vi "雷达流速仪设置窗口.vi"() -> (3 "确定输出":bool)   [LabVIEW 2016, in "雷达流速仪.lvlib"]
panel:
  out "开关":bool
  in  "雷达流速仪类型":string(combo)
  in  "串口":refnum<visa-resource-name>="COM6"
  in  "雷达流速仪型号":string="LDH20-1QC"
  in  "确定":bool
  in  "取消":bool
  in  "串口开关":bool
  # "设置雷达流速仪参数"
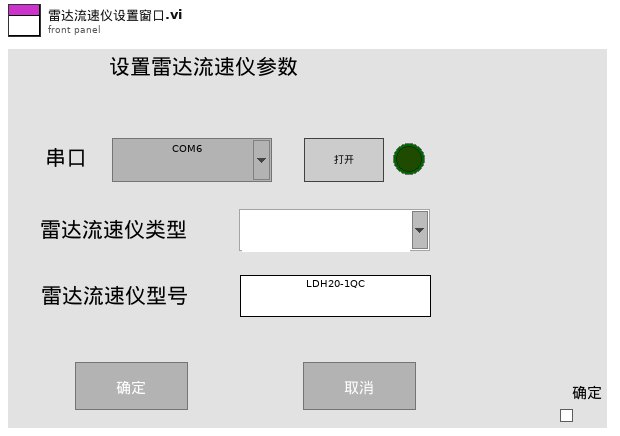
[diagram p1: front panel]
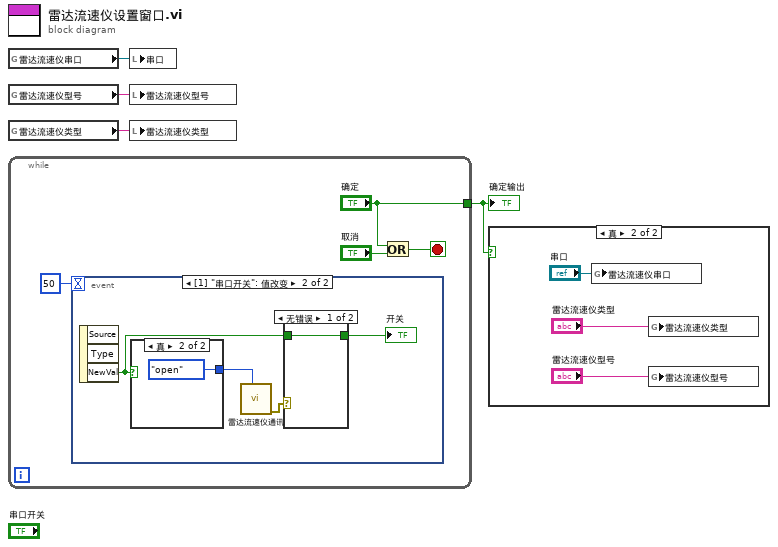
[diagram p0: block diagram]
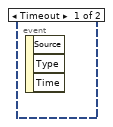
[diagram p3: hidden frame]
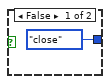
[diagram p5: hidden frame]
diagram:
  n1 = global read "雷达流速仪全局变量.vi" "雷达流速仪串口"() -> (w3:refnum<visa-resource-name>)
  n2 = global read "雷达流速仪全局变量.vi" "雷达流速仪型号"() -> (w2:string)
  n3 = global read "雷达流速仪全局变量.vi" "雷达流速仪类型"() -> (w1:string)
  n4 = while {
    tunnel: ["确定"] -> w4
    stop <- w7 stop-if-true
    n5 = event shown="[1] \"串口开关\": 值改变" {
      selector: _ -> [_ _]
      dyn-events: _ -> [_ _]
      timeout: 50 -> [_ _]
      event Timeout {
        n6 = event-data() -> ()  [unwired: 1 in, 3 out]
      }
      event "串口开关": Value Change {
        n7 = event-data() -> ("NewVal"=w10:bool)  [unwired: 1 in, 2 out]
        n8 = case shown="真" w10 {
          tunnel: [enum16{"open", "read", "write", "close"}."close" ("STEP") enum16{"open", "read", "write", "close"}."open" ("STEP")] -> w12
          frame False {
          }
          frame True {
          }
        }
        n9 = call "雷达流速仪通讯.vi"("STEP"=w12) -> ("error out"=w11:errorcluster)  [unwired: 8 in, 2 out]
        n10 = case shown="无错误" w11 {
          tunnel: w10 -> [w13 _]
          tunnel: [w13 _] -> w9
          frame No Error {
          }
          frame Error {
          }
        }
        "开关" <- w9
      }
    }
    n11 = Or(x="确定", y="取消") -> (x .or. y?=w7:bool)
  }
  "确定输出" <- w4
  n12 = local write "串口"(w3) -> ()
  n13 = local write "雷达流速仪型号"(w2) -> ()
  n14 = local write "雷达流速仪类型"(w1) -> ()
  n15 = case shown="真" w4 {
    frame False {
    }
    frame True {
      n16 = global write "雷达流速仪全局变量.vi" "雷达流速仪串口"("串口") -> ()
      n17 = global write "雷达流速仪全局变量.vi" "雷达流速仪类型"("雷达流速仪类型") -> ()
      n18 = global write "雷达流速仪全局变量.vi" "雷达流速仪型号"("雷达流速仪型号") -> ()
    }
  }
